vi "Default volues.vi"() -> ()   [LabVIEW 2017]
panel:
  in  "CI Settings":T1={"Counter"="Dev1/ctr0", "A Input Terminal"="PFI8", "B Input Terminal"="PFI10", "Pulses Per Revolution"=24, "Z Index Enable"=FALSE, "Z Index Terminal"="PFI9", "Sample Clock Source"="PFI0", "Sample Rate"=1000.0, "Samples per Loop"=100, "Digital Trigger Source"="", "Edge"=10280} {"Edge" items=["Rising"=10280, "Falling"=10171]}
  in  "CO Settings":T2={"Counter"="Dev1/ctr0", "Output Terminal"="/Dev1/PFI12", "source of ticks"="OnboardClock", "high ticks"=100, "low ticks"=100, "Digital Trigger Source"="", "Edge"=10280} {"Edge" items=["Rising"=10280, "Falling"=10171]}
  in  "AI Settings":T3={"AI Channel"="Dev1/ai0", "Min Voltage"=-5.0, "Max Voltage"=5.0, "Terminal Configuration"=-1, "Sample Rate"=1000.0, "Number of Samples"=100, "Logging Mode"=10231, "TDMS File Path"=path "", "Digital Start Trigger Source"="/Dev1/PFI0", "Digital Start Trigger Edge"=10280} {"Digital Start Trigger Edge" items=["Rising"=10280, "Falling"=10171]; "Logging Mode" items=["Off"=10231, "Log and Read"=15842]; "Terminal Configuration" items=["default"=-1, "RSE"=10083, "NRSE"=10078, "Differential"=10106, "Pseudodifferential"=12529]}
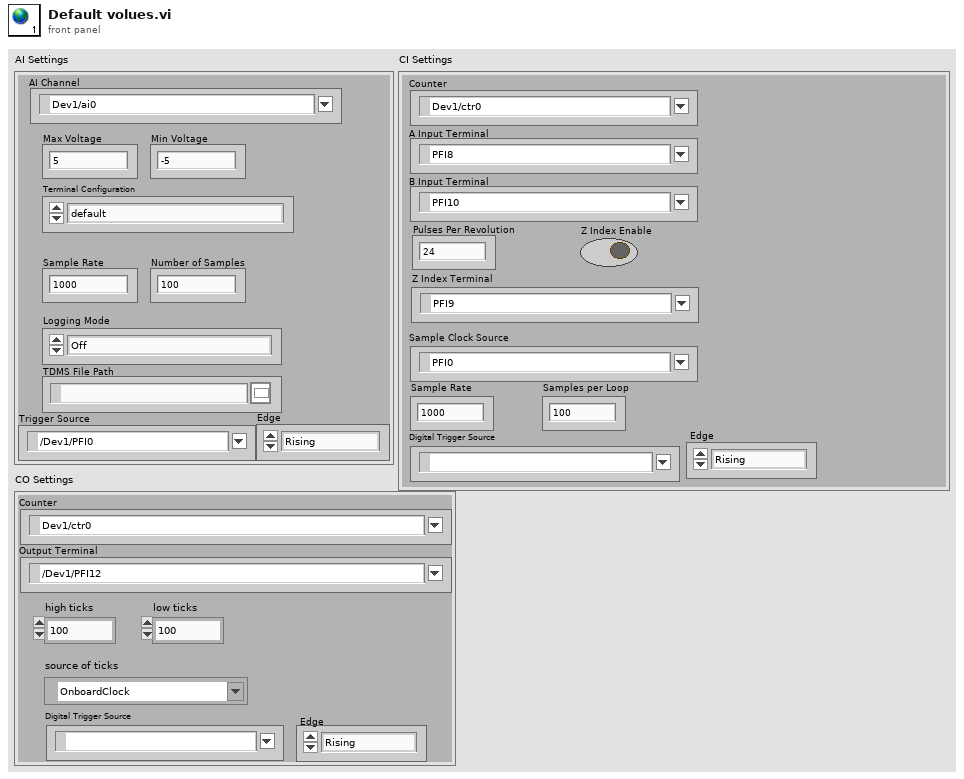
[diagram p1: front panel]
types:
  T1 = cluster{"Counter":tag, "A Input Terminal":tag, "B Input Terminal":tag, "Pulses Per Revolution":u32, "Z Index Enable":bool, "Z Index Terminal":tag, "Sample Clock Source":tag, "Sample Rate":dbl, "Samples per Loop":i32, "Digital Trigger Source":tag, "Edge":i32}
  T2 = cluster{"Counter":tag, "Output Terminal":tag, "source of ticks":tag, "high ticks":u32, "low ticks":u32, "Digital Trigger Source":tag, "Edge":i32}
  T3 = cluster{"AI Channel":tag, "Min Voltage":dbl, "Max Voltage":dbl, "Terminal Configuration":i32, "Sample Rate":dbl, "Number of Samples":i32, "Logging Mode":i32, "TDMS File Path":path, "Digital Start Trigger Source":tag, "Digital Start Trigger Edge":i32}
diagram:
